vi "Phsae_shift_test(2).vi"() -> ()   [LabVIEW 2017]
uses:
  <vilib>/Analysis/3filter.llb/Filter Passband Type.ctl
  <vilib>/Analysis/4window.llb/windowTd.ctl
  <vilib>/Analysis/3filter.llb/FIR Windowed Filter (DBL).vi
  <vilib>/Analysis/NI_AALBase.lvlib
  <vilib>/Analysis/NI_AALPro.lvlib
panel:
  out "SIF0+SIF1":waveform(dbl)(graph)
  in  "Message Signal Phsae":dbl=90.0
  in  "Carrier Frequency(Hz)":dbl=560000.0
  in  "Frequency(Hz)":dbl=600000.0
  in  "Amplitude(Vpeak)":dbl=1.0
  in  "Pulse length(sec)":dbl=0.5
  in  "Sampling frequency(Hz)":dbl=3000000.0
  in  "Delay time.A.1(sec)":dbl=0.5
  out "S0 LPF out FFT(amplitude)":waveform(dbl)(graph)
  out "S1 LPF out FFT(amplitude)":waveform(dbl)(graph)
  out "S1 LPF output":waveform(dbl)(graph)
  out "S0 LPF output":waveform(dbl)(graph)
  out "S0 FFT(amplitude)":waveform(dbl)(graph)
  out "S1 FFT(amplitude) 2":waveform(dbl)(graph)
  out "크기":i32
  out "S0 signal":waveform(dbl)(graph)
  out "S1 signal":waveform(dbl)(graph)
  out "Pulse SIG":dbl[](array[numeric])
  out "Delay SIG.A.1":dbl[](array[numeric])
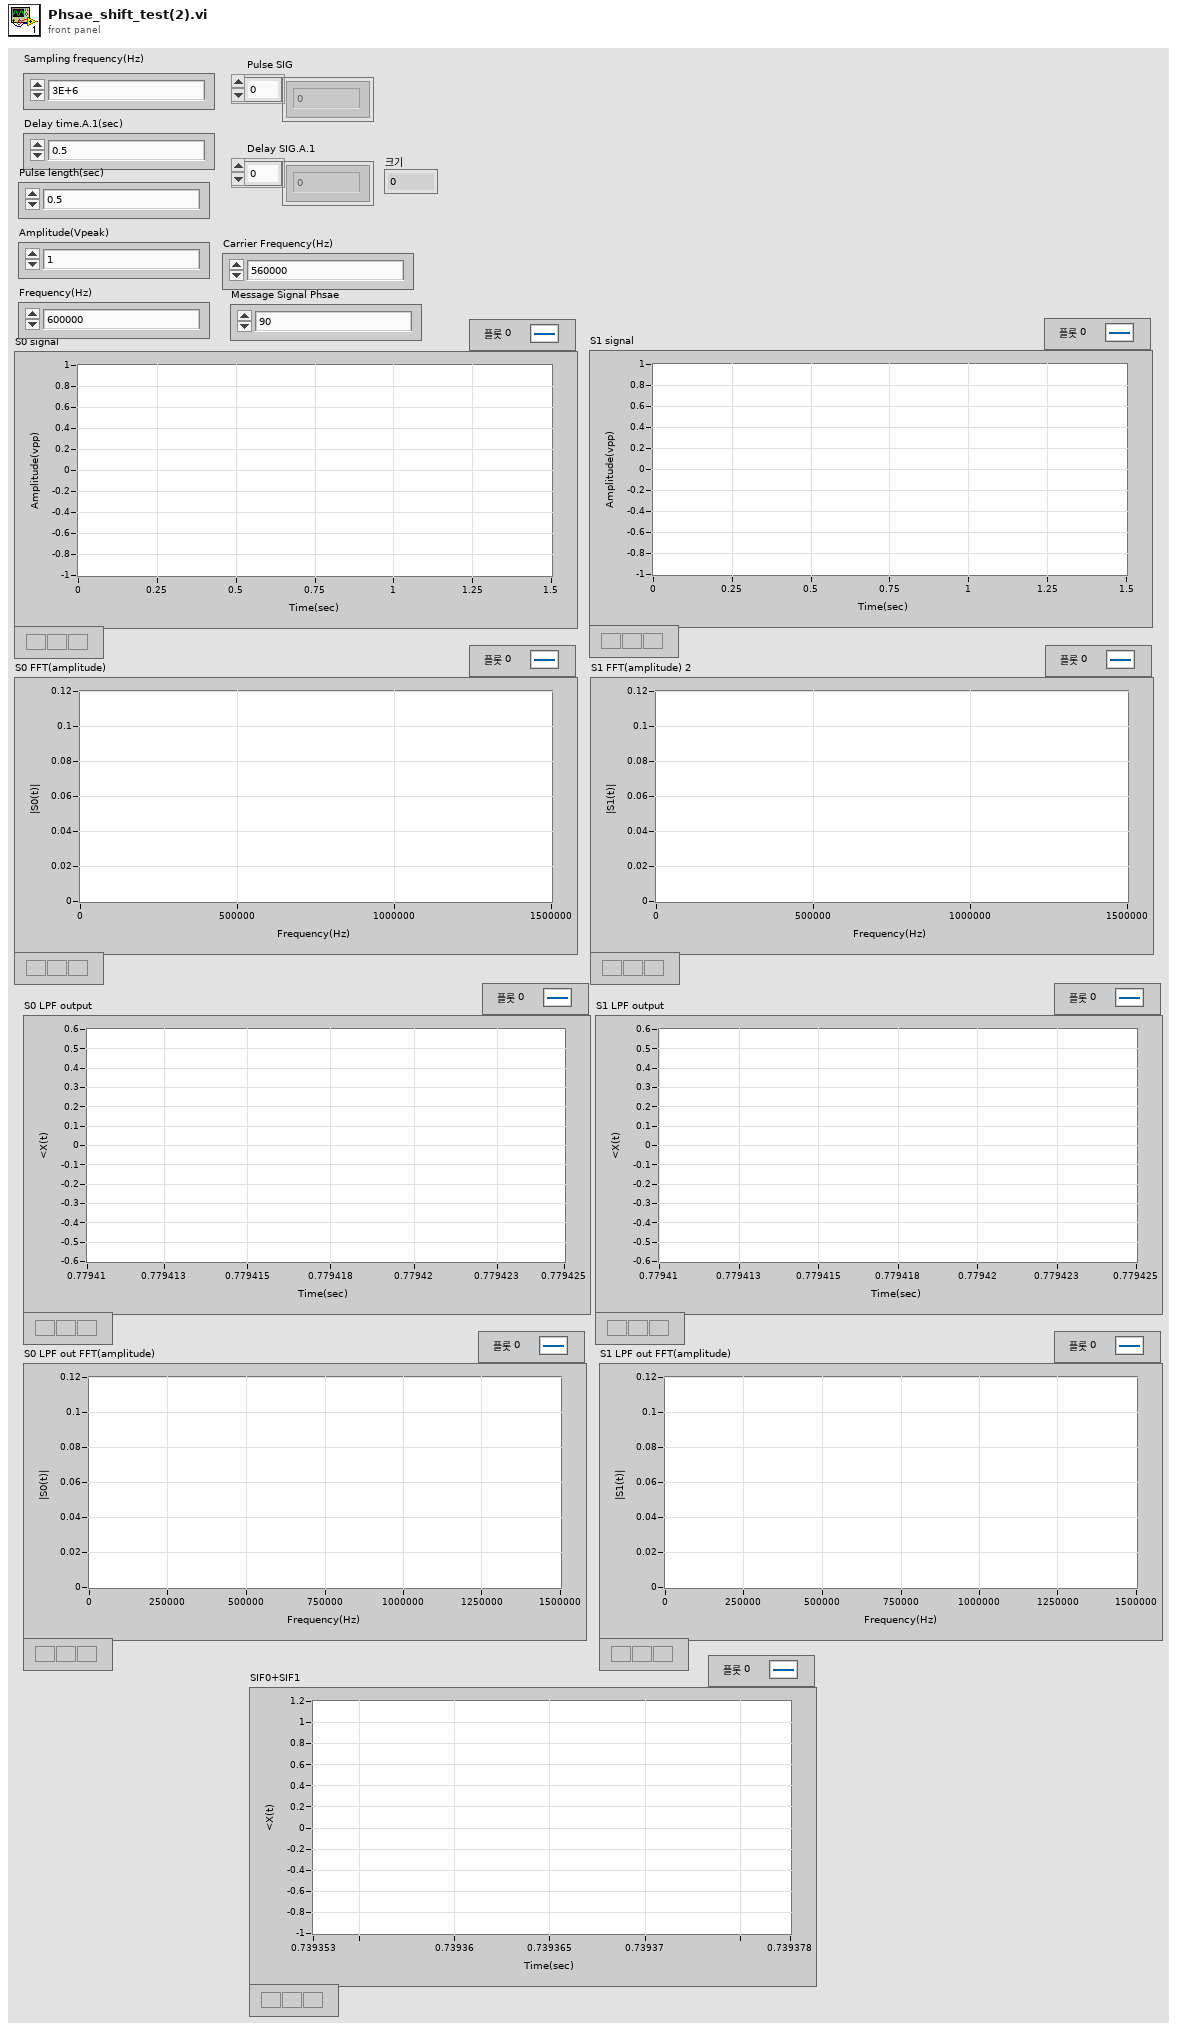
[diagram p1: front panel]
types:
  T1 = typedef "NI_AALBase.lvlib/Filter Passband Type.ctl" = enum32{"Lowpass", "Highpass", "Bandpass", "Bandstop"}
  T2 = typedef "NI_AALPro.lvlib/windowTd.ctl" = u32
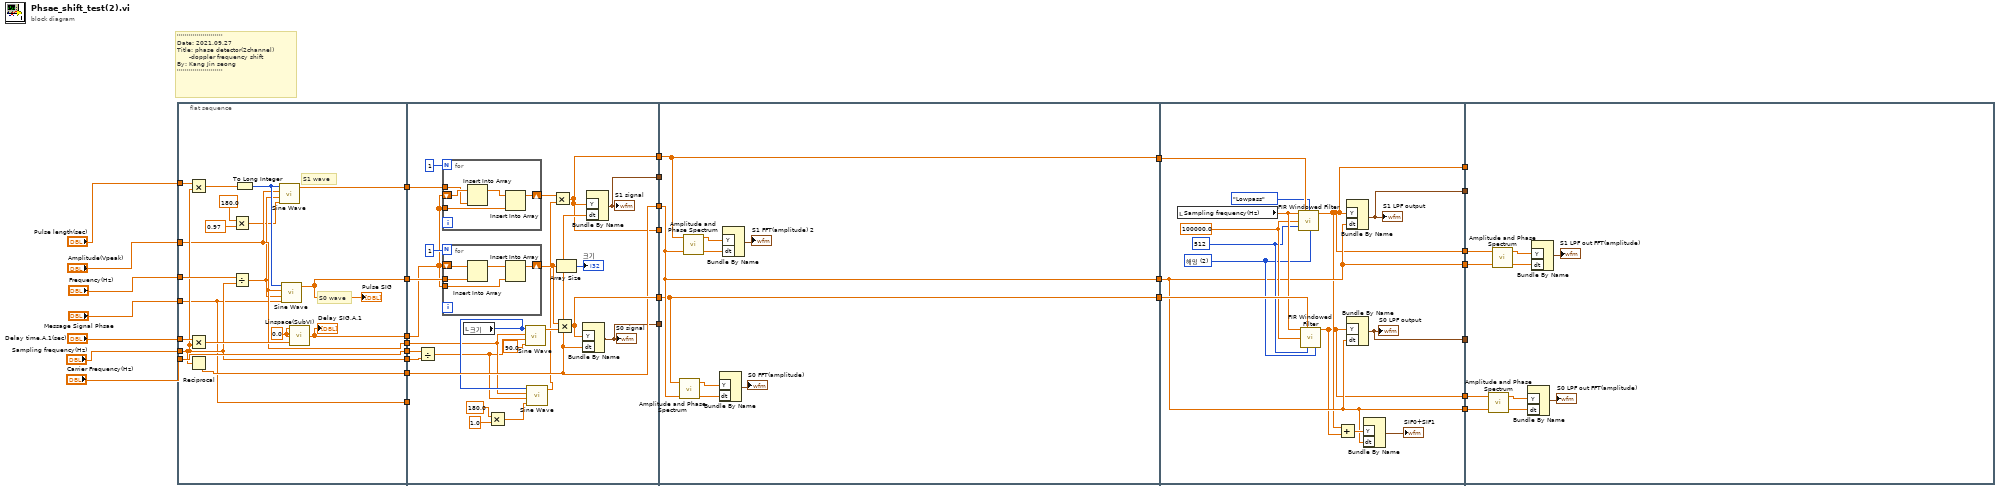
[diagram p0: block diagram]
diagram:
  # "'''''''''''''''''''''''\nDate: 2021.09.27\nTitle: phase detector(2channel)\n      -doppler frequency shift\nBy: Kang Jin seong\n'''''''''''''''''''''''"
  n1 = flat-sequence {
    tunnel: "Frequency(Hz)" -> [w47]
    tunnel: "Amplitude(Vpeak)" -> [w38]
    tunnel: "Pulse length(sec)" -> [w46]
    tunnel: "Sampling frequency(Hz)" -> [w41]
    tunnel: "Delay time.A.1(sec)" -> [w45]
    tunnel: [w40] -> w31
    tunnel: [w44] -> w30
    tunnel: [w43] -> w29
    tunnel: [w38] -> w28
    tunnel: "Carrier Frequency(Hz)" -> [w42]
    tunnel: [w42] -> w27
    tunnel: [w41] -> w26
    tunnel: [w36] -> w25
    tunnel: "Message Signal Phsae" -> [w35]
    tunnel: [w35] -> w2
    tunnel: w31 -> [w73]
    tunnel: w30 -> [w65]
    tunnel: w29 -> [w61]
    tunnel: w28 -> [w56]
    tunnel: w27 -> [w70]
    tunnel: w26 -> [w69]
    tunnel: w25 -> [w66]
    tunnel: [w60] -> w22
    tunnel: [w61] -> w23
    tunnel: [w62] -> w24
    tunnel: [w60] -> w21
    tunnel: [w59] -> w20
    tunnel: [w58] -> w19
    tunnel: w2 -> [_]
    tunnel: w24 -> [w85]
    tunnel: w23 -> [w86]
    tunnel: w22 -> [w88]
    tunnel: w21 -> [_]
    tunnel: w20 -> [_]
    tunnel: w19 -> [_]
    tunnel: [w88] -> w18
    tunnel: [w86] -> w17
    tunnel: [w85] -> w16
    tunnel: w18 -> [w107]
    tunnel: w17 -> [w97]
    tunnel: w16 -> [w105]
    tunnel: [w100] -> w15
    tunnel: [w95] -> w14
    tunnel: [w97] -> w13
    tunnel: [w99] -> w12
    tunnel: [w94] -> w11
    tunnel: [w97] -> w10
    tunnel: [w95] -> w1
    tunnel: w15 -> [_]
    tunnel: w14 -> [w112]
    tunnel: w13 -> [w111]
    tunnel: w12 -> [_]
    tunnel: w11 -> [w109]
    tunnel: w10 -> [w110]
    tunnel: w1 -> [_]
    frame #0 {
      w48 = 0.0 ("frequency")
      # "S1 wave"
      # "S0 wave"
      n2 = Multiply(x=w46, y=w41) -> (x*y=w50:dbl)
      n3 = Multiply(x=w45, y=w41) -> (x*y=w49:dbl)
      n4 = Reciprocal(x=w41) -> (1/x=w43:dbl)
      n5 = Multiply(x=180.0 ("phase in"), y=0.97) -> (x*y=w32:dbl)
      n6 = Divide(x=w47, y=w41) -> (x/y=w37:dbl)
      n7 = To Long Integer(number=w50) -> (32bit integer=w39:i32)
      n8 = call <vilib>:"Sine Wave.vi"("samples"=w39, "amplitude"=w38, "frequency"=w37, "phase in"=w32) -> ("sine wave"=w36:dbl[])  [unwired: 1 in, 2 out]
      n9 = call <vilib>:"Sine Wave.vi"("samples"=w39, "amplitude"=w38, "frequency"=w37, "phase in"=w35) -> ("sine wave"=w40:dbl[])  [unwired: 1 in, 2 out]
      "Pulse SIG" <- w40
      n10 = call "Linspace(SubVI).vi"("NumElements"=w49, "End"=w48, "Start"=w48) -> ("Array"=w44:dbl[])
      "Delay SIG.A.1" <- w44
    }
    frame #1 {
      n11 = Divide(x=w70, y=w69) -> (x/y=w55:dbl)
      n12 = for {
        N: 1 -> [_]
        shift-right: [w75] -> w64
        shift-left: w65 -> [w79]
        tunnel: w66 -> [w78]
        tunnel: w65 -> [w76]
        n13 = Insert Into Array(array=w79, new element=w78) -> (w77:dbl[])  [unwired: 1 in]
        n14 = Insert Into Array(array=w77, new element=w76) -> (w75:dbl[])  [unwired: 1 in]
      }
      n15 = for {
        N: 1 -> [_]
        shift-right: [w80] -> w68
        shift-left: w65 -> [w84]
        tunnel: w73 -> [w83]
        tunnel: w65 -> [w81]
        n16 = Insert Into Array(array=w84, new element=w83) -> (w82:dbl[])  [unwired: 1 in]
        n17 = Insert Into Array(array=w82, new element=w81) -> (w80:dbl[])  [unwired: 1 in]
      }
      n18 = local read "크기"() -> (w57:i32)
      n19 = Multiply(x=180.0 ("phase in"), y=1.0) -> (x*y=w52:dbl)
      n20 = call <vilib>:"Sine Wave.vi"("samples"=w57, "amplitude"=w56, "frequency"=w55, "phase in"=90.0) -> ("sine wave"=w63:dbl[])  [unwired: 1 in, 2 out]
      n21 = call <vilib>:"Sine Wave.vi"("samples"=w57, "amplitude"=w56, "frequency"=w55, "phase in"=w52) -> ("sine wave"=w54:dbl[])  [unwired: 1 in, 2 out]
      n22 = Multiply(x=w64, y=w54) -> (x*y=w60:dbl[])
      n23 = Multiply(x=w68, y=w63) -> (x*y=w62:dbl[])
      n24 = Array Size(array=w68) -> (size(s)=→"크기":i32)
      n25 = Bundle By Name("Y"=w62, "dt"=w61) -> (w59:waveform(dbl))  [unwired: 1 in]
      "S0 signal" <- w59
      n26 = Bundle By Name("Y"=w60, "dt"=w61) -> (w58:waveform(dbl))  [unwired: 1 in]
      "S1 signal" <- w58
    }
    frame #2 {
      n27 = call <vilib>:"Amplitude and Phase Spectrum.vi"("dt"=w86, "Signal (V)"=w85) -> ("df"=w91:dbl, "Amp Spectrum Mag (Vrms)"=w93:dbl[])  [unwired: 1 in, 1 out]
      n28 = call <vilib>:"Amplitude and Phase Spectrum.vi"("dt"=w86, "Signal (V)"=w88) -> ("df"=w87:dbl, "Amp Spectrum Mag (Vrms)"=w90:dbl[])  [unwired: 1 in, 1 out]
      n29 = Bundle By Name("Y"=w93, "dt"=w91) -> (→"S0 FFT(amplitude)":waveform(dbl))  [unwired: 1 in]
      n30 = Bundle By Name("Y"=w90, "dt"=w87) -> (→"S1 FFT(amplitude) 2":waveform(dbl))  [unwired: 1 in]
    }
    frame #3 {
      w101 = T2 2 items=["사각형"=0, "해닝"=1, "해밍"=2, "블랙맨-해리스"=3, "정밀한 블랙맨"=4, "블랙맨"=5, "플랫 탑"=6, "4항 블랙맨-해리스 "=7, "7항 블랙맨-해리스"=8, "낮은 사이드로브"=9, "블랙맨 누탈"=11, "삼각형"=30, "바틀렛-해닝"=31, "보먼"=32, "파젠"=33, "웰치"=34, "카이저"=60, "돌프-체비셰프"=61, "가우스"=62] ("window")
      w102 = 512 ("taps")
      w103 = 100000.0 ("low cutoff freq: fl")
      n31 = local read "Sampling frequency(Hz)"() -> (w104:dbl)
      n32 = call-poly <vilib>:"FIR Windowed Filter.vi"("sampling freq: fs"=w104, "X"=w107, "filter type"=Filter_Passband_Type."Lowpass", "low cutoff freq: fl"=w103, "taps"=w102, "window"=w101) -> ("Filtered X"=w95:dbl[])  [unwired: 8 in, 1 out]
      n33 = call-poly <vilib>:"FIR Windowed Filter.vi"("sampling freq: fs"=w104, "X"=w105, "low cutoff freq: fl"=w103, "taps"=w102, "window"=w101) -> ("Filtered X"=w94:dbl[])  [unwired: 9 in, 1 out]
      n34 = Add(x=w95, y=w94) -> (x+y=w98:dbl[])
      n35 = Bundle By Name("Y"=w95, "dt"=w97) -> (w100:waveform(dbl))  [unwired: 1 in]
      "S1 LPF output" <- w100
      n36 = Bundle By Name("Y"=w94, "dt"=w97) -> (w99:waveform(dbl))  [unwired: 1 in]
      "S0 LPF output" <- w99
      n37 = Bundle By Name("Y"=w98, "dt"=w97) -> (→"SIF0+SIF1":waveform(dbl))  [unwired: 1 in]
    }
    frame #4 {
      n38 = call <vilib>:"Amplitude and Phase Spectrum.vi"("dt"=w110, "Signal (V)"=w109) -> ("df"=w115:dbl, "Amp Spectrum Mag (Vrms)"=w117:dbl[])  [unwired: 1 in, 1 out]
      n39 = call <vilib>:"Amplitude and Phase Spectrum.vi"("dt"=w111, "Signal (V)"=w112) -> ("df"=w108:dbl, "Amp Spectrum Mag (Vrms)"=w114:dbl[])  [unwired: 1 in, 1 out]
      n40 = Bundle By Name("Y"=w117, "dt"=w115) -> (→"S0 LPF out FFT(amplitude)":waveform(dbl))  [unwired: 1 in]
      n41 = Bundle By Name("Y"=w114, "dt"=w108) -> (→"S1 LPF out FFT(amplitude)":waveform(dbl))  [unwired: 1 in]
    }
  }
